vi "Element Type.vi"(11 "2WayValve in":refnum<class "2WayValveH.lvclass">) -> (2 "Control Type":string)   [LabVIEW 2020, in "VolatusGUIElements.lvlib" / "2WayValveH.lvclass"]
uses:
  2WayValveH.lvclass
  2WayValveH.lvclass/2WayValveH.ctl
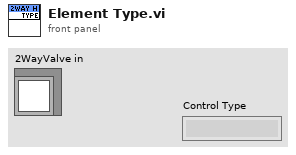
[diagram p1: front panel]
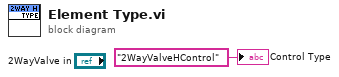
[diagram p0: block diagram]
diagram:
  "Control Type" <- "2WayValveHControl" ("Control Type")
